vi "Host_Main - STM.vi"() -> ()   [LabVIEW 2014]
uses:
  <vilib>/NI/STM/SubVIs/MetaDataElement.ctl
  <vilib>/NI/STM/TCP/TCP Read Options.ctl
  <vilib>/NI/STM/TCP/Read Meta Data (TCP Ref).vi
  <vilib>/NI/STM/TCP/Get Connection Reference (TCP).vi
  <vilib>/NI/STM/TCP/Read Meta Data (TCP Clst).vi
  <vilib>/NI/STM/TCP/Read Message (TCP).vi
  <vilib>/NI/STM/NI STM.lvlib
panel:
  out "name":T1
  in  "stop":bool
  out "Waveform Graph":cluster{"f0":dbl, "df":dbl, "magnitude":dbl[]}(graph)
  out "error  out":errorcluster
  in  "Target IP Address":string="192.168.2.52"
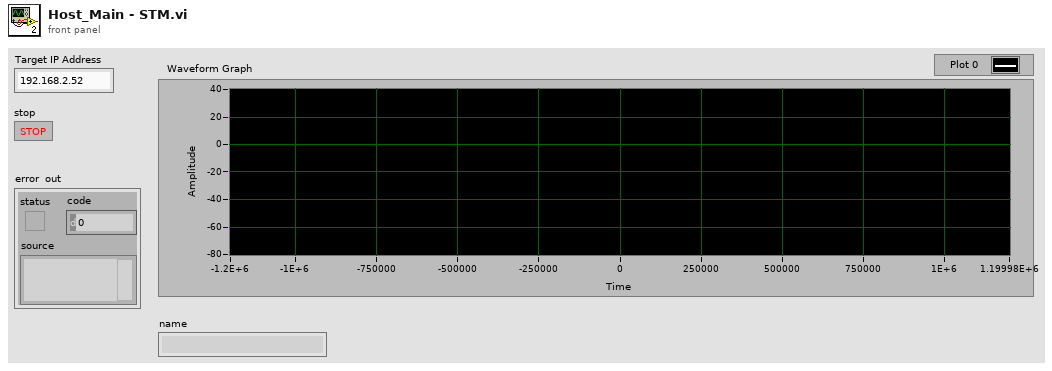
[diagram p1: front panel]
types:
  T1 = typedef "NI STM.lvlib/MetaDataElement.ctl" = string
  T2 = typedef "NI STM.lvlib/TCP Connection Info.ctl" = cluster{"connection ID":refnum<k5>, "meta data":T1[]}
  T3 = typedef "NI STM.lvlib/TCP Read Options.ctl" = cluster{"ignore timeout error":bool, "timeout ms (1000)":i32}
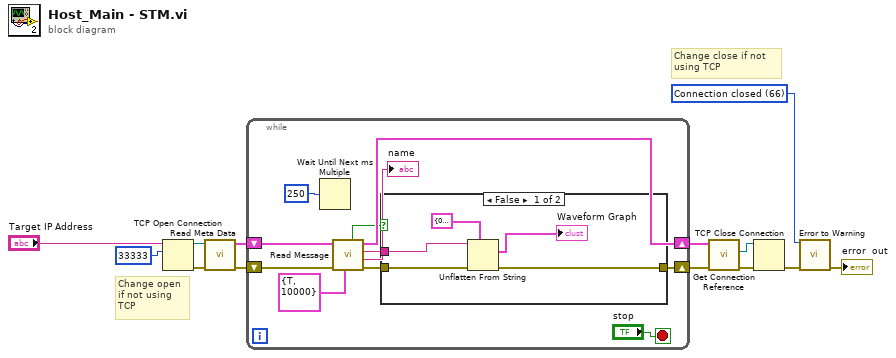
[diagram p0: block diagram]
diagram:
  w11 = 66 items=["No Error", "Argument Error", "Memory Full", "Out of Zone", "End of File", "File Already Open", "Generic File IO Error", "File Not Found", "File Permission Error", "Disk Full", "Duplicate Path", "Too Many Files Open", "Not Enabled", "Resource File Not Found", "Cannot Add Resource", "Resource Not Found", "Image Not Found", "Image Memory Error", "Pen Does Not Exist", "Config Bad Type", "Config Token Not Found", "Config Parse Error", "Config Memory Error", "Bad External Code Format", "Bad External Code Offset", "External Code Not Present", "Null Window", "Destroy Window Mixup", "Null Menu", "Print Aborted", "Bad Print Record", "Print Driver Error", "Windows Error During Print", "Memory Error During Print", "Print Dialog Error", "Generic Print Error", "Invalid Device Refnum", "Device Not Found", "Device Parameter Error", "Device Unit Error", "Can't Open Device", "Device Call Aborted", "Generic Error", "Cancelled By User", "Object ID Too Low", "Object ID Too High", "Object Not In Heap", "Unknown Heap", "Bad DefProc ID", "DefProc Not In Table", "Message Out Of Range", "Null Method", "Unknown Message", "Manager Call Not Supported", "Bad address", "Connection In progress", "Connection timed out", "Connection is already in progress", "Network attribute not supported", "Network error", "Address in use", "System out of memory", "Connection aborted", "Connection refused", "Connection is not connected", "Connection is already connected", "Connection closed", "Initialize error (interapplication manager)", "Bad occurrence", "Wait on unbound occurrence handler", "Occurrence queue overflow", "Bad path", "Semaphore not signaled", "Unrecognized type (interapplication manager)"] ("1st Error to Convert")
  # "Change close if not using TCP"
  # "Change open if not using TCP"
  n1 = TCP Open Connection(address="Target IP Address", remote port or service name=u16 33333 ("remote port")) -> (connection ID=w10:refnum<k5>, error out=w9:errorcluster)  [unwired: 1 in, 2 out]
  n2 = call-poly <vilib>:"Read Meta Data.vi"("error in"=w9, "connection ID"=w10) -> ("error out"=w3:errorcluster, "connection info out"=w4:T2)  [unwired: 1 in, 7 out]
  n3 = while {
    shift-right: [w21] -> w2
    shift-left: w4 -> [w24]
    shift-right: [w19] -> w1
    shift-left: w3 -> [w23]
    stop <- "stop" stop-if-true
    n4 = Wait Until Next ms Multiple(millisecond multiple=u32 250) -> ()  [unwired: 1 out]
    n5 = call-poly <vilib>:"Read Message.vi"("options"=T3 {"ignore timeout error"=TRUE, "timeout ms (1000)"=10000}, "error in"=w23, "connection info in"=w24) -> ("error out"=w20:errorcluster, "name"=→"name":T1, "data string"=w18:string, "connection info out"=w21:T2, "timed out?"=w15:bool)  [unwired: 3 in, 1 out]
    n6 = case shown="False" w15 {
      tunnel: w20 -> [w29 w30]
      tunnel: [w28 w30] -> w19
      tunnel: w18 -> [w27 _]
      frame False {
        n7 = Unflatten From String(type=cluster{"f0":dbl, "df":dbl, "magnitude":dbl[]} {"f0"=0.0, "df"=0.0, "magnitude"=[]} ("element"), binary string=w27, error in (no error)=w29) -> (value=→"Waveform Graph":cluster{"f0":dbl, "df":dbl, "magnitude":dbl[]}, error out=w28:errorcluster)  [unwired: 2 in, 1 out]
      }
      frame True {
      }
    }
  }
  n8 = call-poly <vilib>:"Get Connection Reference.vi"("error in"=w1, "connection info in"=w2) -> ("error out"=w6:errorcluster, "connection ID out"=w5:refnum<k5>)  [unwired: 8 out]
  n9 = TCP Close Connection(connection ID=w5, error in (no error)=w6) -> (error out=w12:errorcluster)  [unwired: 2 out]
  n10 = call <vilib>:"Error to Warning.vi"("1st Error to Convert"=w11, "error in"=w12) -> ("warning out"=→"error  out":errorcluster)  [unwired: 3 in, 10 out]
